vi "Parse Authority.vi"(10 "error in (no error)":errorcluster, 11 "Authority String":string) -> (2 "error out":errorcluster, 3 "Authority":T1)   [LabVIEW 2020, in "URI.lvlib"]
uses:
  URI.lvlib
  Authority.ctl
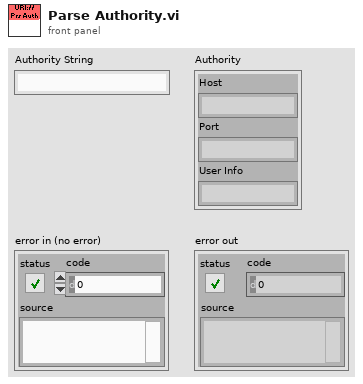
[diagram p1: front panel]
types:
  T1 = typedef "URI.lvlib/Authority.ctl" = cluster{"Host":string, "Port":string, "User Info":string}
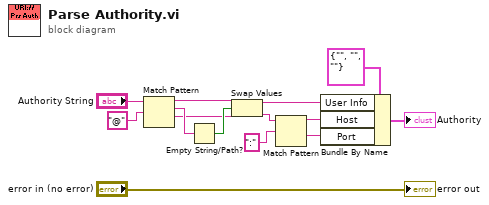
[diagram p0: block diagram]
diagram:
  n1 = Match Pattern(string="Authority String", regular expression="@") -> (before substring=w12:string, match substring=w14:string, after substring=w11:string)  [unwired: 1 in, 1 out]
  n2 = Empty String/Path?(string/path=w14) -> (empty?=w13:bool)
  n3 = Swap Values(12:w12, 13:w13, 14:w11) -> (1:w4:string, 3:w9:string)
  n4 = Match Pattern(string=w9, regular expression=":") -> (before substring=w3:string, after substring=w2:string)  [unwired: 1 in, 2 out]
  n5 = Bundle By Name(cluster=T1 {"Host"="", "Port"="", "User Info"=""} ("Authority"), "User Info"=w4, "Host"=w3, "Port"=w2) -> (→"Authority":T1)
  "error out" <- "error in (no error)"
